vi "AI Interrupt Handling.vi"() -> ()   [LabVIEW 2021]
uses:
  <vilib>/myRIO/Instrument Drivers/Utilities/Utilities.lvlib
  <vilib>/Platform/TimedLoop/XDataNode/wakeup.ctl
  <vilib>/Platform/TimedLoop/XDataNode/XDNodeRunTimeDep.lvlib
  <vilib>/Platform/TimedLoop/XDataNode/nitl_modes.ctl
  <vilib>/Platform/TimedLoop/XDataNode/timing_clust.ctl
  <vilib>/Platform/TimedLoop/XDataNode/XDataNode.xnode
  <vilib>/myRIO/Express VI/IRQ/IRQ Express VI.xnode
  <vilib>/myRIO/Common/Instrument Driver Framework/myRIO v1.0/IRQ/typedefs/AI IRQ Type.ctl
  <vilib>/myRIO/Common/Instrument Driver Framework/myRIO v1.0/IRQ/typedefs/Callback VI Ref.ctl
  <vilib>/myRIO/Instrument Drivers/IRQ/IO IRQ/vis/myRIO Register AI IRQ.xnode
  <vilib>/myRIO/Common/Instrument Driver Framework/myRIO v1.0/IRQ/vis/myRIO v1.1 Register AI IRQ.vi
  <vilib>/userdefined/High Color/nirio_resource_hc.ctl
  AI Callback 1 CPU.vi
  AI Callback 2 CPUs.vi
  <vilib>/myRIO/Express VI/Onboard IO/AI/AI Express VI.xnode
  <vilib>/myRIO/Instrument Drivers/Onboard IO/AI/vis/Read.vi
  <vilib>/myRIO/Instrument Drivers/Onboard IO/AI/AI.lvlib
  <vilib>/myRIO/Common/Instrument Driver Framework/Utilities/typedefs/Analog Scaling Constants.ctl
  <vilib>/myRIO/Common/Instrument Driver Framework/Utilities/typedefs/Analog Scaling Constants List.ctl
  <vilib>/myRIO/Common/Instrument Driver Framework/myRIO v1.0/AI/typedefs/AI Channels Enum.ctl
  <vilib>/myRIO/Common/Instrument Driver Framework/myRIO v1.0/AI/typedefs/AI Channels List.ctl
  <vilib>/myRIO/Common/Instrument Driver Framework/Utilities/typedefs/Generic FPGA Reference.ctl
  <vilib>/myRIO/Common/Instrument Driver Framework/Utilities/typedefs/myRIO v1.0 Reference.ctl
  <vilib>/myRIO/Common/Instrument Driver Framework/Utilities/typedefs/Hardware Version Enum.ctl
  <vilib>/myRIO/Common/Instrument Driver Framework/Utilities/typedefs/myRIO Generic Hardware Reference.ctl
  <vilib>/myRIO/Instrument Drivers/Onboard IO/AI/typedefs/AI Reference.ctl
  <vilib>/myRIO/Instrument Drivers/Onboard IO/AI/vis/myRIO AI Open.xnode
  <vilib>/myRIO/Common/Instrument Driver Framework/Utilities/vis/Is FPGA Ref Available.vi
  <vilib>/myRIO/Common/Instrument Driver Framework/myRIO v1.0/AI/vis/myRIO v1.1 Open AI.vi
panel:
  out "error out":errorcluster
  in  "Mode":T1(ring)
  out "Waveform Chart":cluster{"A/AI0 (Pin 3)":dbl, "element":dbl}(graph)
  in  "stop":bool
  # "Overview: This VI demonstrates how to use callback VIs handle an analog input interrupt.\nInstructions:\n1.\tConnect an external analog signal to the A/AI0 (Pin 3) with a cable. A/ stands for connector A on the myRIO.\n2.\tIn the Project Explorer window, verify the IP address of the myRIO target. If it is incorrect, update the IP address.\n3.\tRun the VI.\n4.\tThe waveform displays the analog input signal that the VI reads on the AI0 channel.\n5.\tThe threshold for triggering the analog input is 4 V. The VI triggers an interrupt on the rising edge of the analog input signal. Thus, every time when the analog input signal meets both prerequisites, an impulse appears on the trigger point in the waveform chart.\n6.\tThe VI includes two callback VIs. One VI uses one CPU, whereas the other VI uses two CPUs. To see the different impacts between the two modes, change the value of Mode."
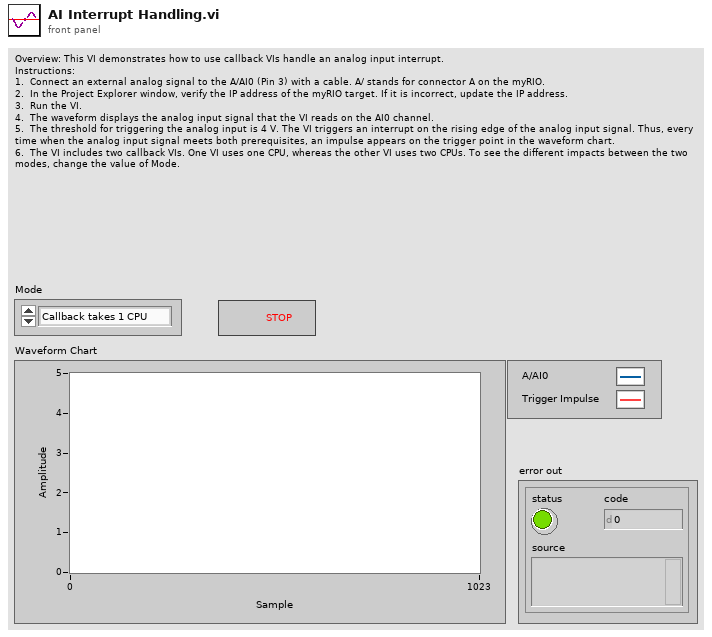
[diagram p1: front panel]
types:
  T1 = enum16{"Callback takes 1 CPU", "Callback takes 2 CPUs"}
  T2 = typedef "AI IRQ Type.ctl" = enum16{"Analog falling edge", "Analog rising edge"}
  T3 = typedef "nirio_resource_hc.ctl" = tag
  T4 = typedef "AI.lvlib/AI Reference.ctl" = cluster{"myRIO Reference":T5, "AI Channels List":T9, "AI Scaling Constants List":T11}
  T5 = typedef "myRIO Generic Hardware Reference.ctl" = cluster{"myRIO Model":T6, "myRIO Hardware Reference":T7}
  T6 = typedef "Hardware Version Enum.ctl" = enum16{"Unknown", "myRIO-1900", "myRIO-1950", "roboRIO", "NI ELVIS RIO CM", "ELVIS III"}
  T7 = typedef "myRIO v1.0 Reference.ctl" = cluster{"Generic FPGA Reference":T8, "Allow multiple opens":bool}
  T8 = typedef "Generic FPGA Reference.ctl" = refnum<k20>
  T9 = typedef "AI Channels List.ctl" = T10[]
  T10 = typedef "AI Channels Enum.ctl" = enum16{"Not Connected", "AudioIn/Left", "AudioIn/Right", "C/AI0", "C/AI1", "A/AI0", "A/AI1", "A/AI2", "A/AI3", "A/AI4", "A/AI5", "A/AI6", "A/AI7", "B/AI0", "B/AI1", "B/AI2", "B/AI3", "B/AI4", "B/AI5", "B/AI6", "B/AI7", "AI/AI0", "AI/AI1", "AI/AI2", "AI/AI3", "A/AI0 (DIFF)", "A/AI1 (DIFF)", "A/AI2 (DIFF)", "A/AI3 (DIFF)", "B/AI0 (DIFF)", "B/AI1 (DIFF)", "B/AI2 (DIFF)", "B/AI3 (DIFF)"}
  T11 = typedef "Analog Scaling Constants List.ctl" = T12[]
  T12 = typedef "Analog Scaling Constants.ctl" = cluster{"LSB Weight (Volts)":dbl, "Offset (Volts)":dbl, "Signed?":bool}
  T13 = typedef "XDNodeRunTimeDep.lvlib/timing_clust.ctl" = cluster{"Expected End [f-1]":u64, "Actual End [f-1]":u64, "Finished Late? [f-1]":bool, "Expected End [i-1]":u64, "Actual End [i-1]":u64, "Finished Late? [i-1]":bool, "Expected Start [i]":u64, "Actual Start [i]":u64, "Expected Start [f]":u64, "Actual Start [f]":u64, "Source Name":string, "Structure Name":string, "Period":i64, "Deadline":i64, "Offset":i64, "Start":i64, "Priority":i32, "Timeout":i32, "Mode":T14, "Wakeup Reason":T15, "Error":errorcluster, "Source Type":string, "Secondary Source Type":string, "Global End Time":u64, "Global Start Time":u64, "Frame Duration":u64, "Iteration Duration":u64, "Assigned CPU":i32, "I/O Scan Engine Mode":u32}
  T14 = typedef "XDNodeRunTimeDep.lvlib/nitl_modes.ctl" = enum32{"No Change", "Process missed periods, maintain original phase", "Discard missed periods, maintain original phase", "Process missed periods, ignore original phase", "Discard missed periods, ignore original phase"}
  T15 = typedef "XDNodeRunTimeDep.lvlib/wakeup.ctl" = enum32{"Normal", "Aborted", "Asynchronous wakeup", "Timing source error", "Timed loop error", "Timeout"}
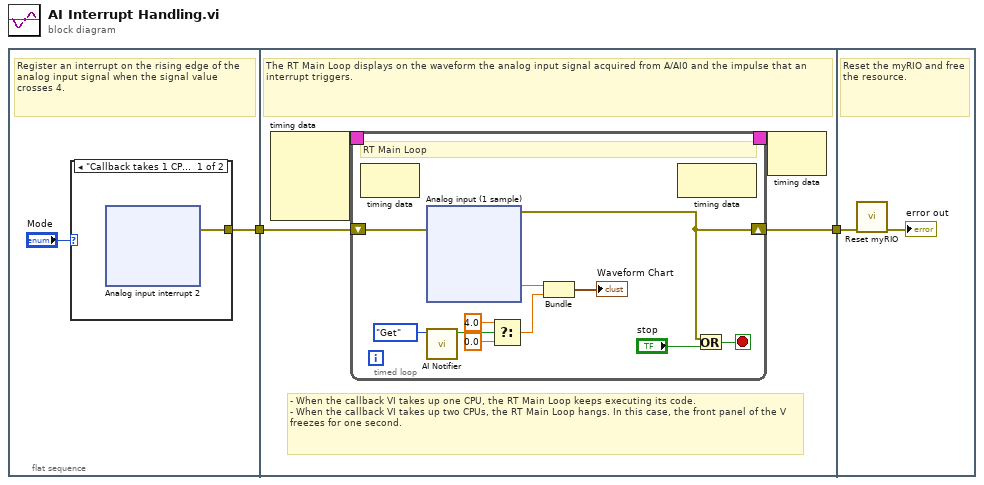
[diagram p0: block diagram]
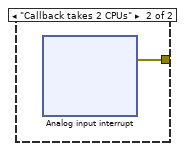
[diagram p2: hidden frame]
diagram:
  n1 = flat-sequence {
    tunnel: [w4] -> w2
    tunnel: w2 -> [w44]
    tunnel: [w43] -> w1
    tunnel: w1 -> [w100]
    frame #0 {
      # "Register an interrupt on the rising edge of the analog input signal when the signal value crosses 4."
      n2 = case shown="\"Callback takes 1 CPU\"" "Mode" {
        tunnel: [w5 w24] -> w4
        frame "Callback takes 1 CPU" {
          n3 = xnode "Analog input interrupt 2"() -> ("error out"=w5:errorcluster)  [unwired: 1 in]
        }
        frame "Callback takes 2 CPUs" {
          n4 = xnode "Analog input interrupt"() -> ("error out"=w24:errorcluster)  [unwired: 1 in]
        }
      }
    }
    frame #1 {
      # "- When the callback VI takes up one CPU, the RT Main Loop keeps executing its code.\n- When the callback VI takes up two CPUs, the RT Main Loop hangs. In this case, the front panel of the V freezes for one second."
      # "The RT Main Loop displays on the waveform the analog input signal acquired from A/AI0 and the impulse that an interrupt triggers."
      n5 = node-c288() -> (w46:T13)  [unwired: 4 in]
      n6 = timed-loop {
        timing: w46 -> [_]
        timing-out: [_] -> w45
        shift-right: [w48] -> w43
        shift-left: w44 -> [w49]
        stop <- w50 stop-if-true
        # "RT Main Loop"
        n7 = node-c288() -> ()  [unwired: 1 in, 1 out]
        n8 = xnode "Analog input (1 sample)"("error in (no error)"=w49) -> ("A/AI0 (Pin 3)"=w47:dbl, "error out"=w48:errorcluster)
        n9 = call "AI Notifier.vi"("Action"=enum16{"Get", "Set"}."Get") -> ("Trigger?"=w56:bool)  [unwired: 10 in]
        n10 = Select(t=4.0 ("element"), s=w56, f=0.0 ("element")) -> (s? t:f=w53:dbl)
        n11 = Bundle("A/AI0 (Pin 3)"=w47, "element"=w53) -> (→"Waveform Chart":cluster{"A/AI0 (Pin 3)":dbl, "element":dbl})  [unwired: 1 in]
        n12 = node-c288() -> ()  [unwired: 1 in, 1 out]
        n13 = Or(x=w48, y="stop") -> (x .or. y?=w50:bool)
      }
      n14 = node-c288(w45) -> ()  [unwired: 1 out]
    }
    frame #2 {
      # "Reset the myRIO and free the resource."
      n15 = call <vilib>:"Reset myRIO.vi"("error in (no error)"=w100) -> ("error out"=→"error out":errorcluster)  [unwired: 10 in]
    }
  }
